vi "Roll Rocks for Platform Tilt.vi"(11 "Array in":u8[](array[numeric])) -> (3 "Array out":u8[](array[numeric]))   [LabVIEW 2022 SP3]
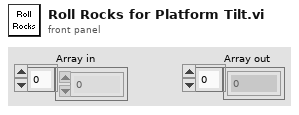
[diagram p1: front panel]
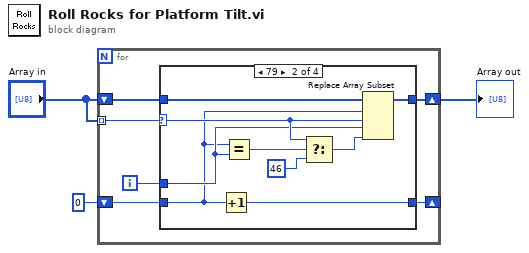
[diagram p0: block diagram]
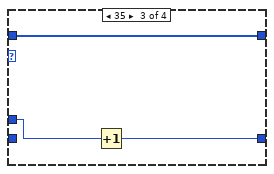
[diagram p3: hidden frame]
diagram:
  n1 = for {
    tunnel: "Array in" -> [w9] mode=indexing
    shift-right: [w7] -> _
    shift-left: 0 -> [w8]
    shift-right: [w5] -> w3
    shift-left: "Array in" -> [w6]
    i -> [w4]
    n2 = case shown="79" w9 {
      selector: w9 -> [_ w16 _ _]
      tunnel: w8 -> [w10 w12 _ w25]
      tunnel: [w10 w20 w22 w25] -> w7
      tunnel: w6 -> [w11 w19 w23 w24]
      tunnel: [w11 w18 w23 w24] -> w5
      tunnel: w4 -> [_ w13 w21 _]
      frame Default {
      }
      frame 79 {
        n3 = Increment(x=w12) -> (x+1=w20:i32)
        n4 = Equal?(x=w12, y=w13) -> (x = y?=w17:bool)
        n5 = Select(t=w16, s=w17, f=u8 46) -> (s? t:f=w14:u8)
        n6 = Replace Array Subset(array=w19, new element #1=w16, index #1=w12, new element #2=w14, index #2=w13) -> (w18:u8[])
      }
      frame 35 {
        n7 = Increment(x=w21) -> (x+1=w22:i32)
      }
      frame 46 {
      }
    }
  }
  "Array out" <- w3
